vi "day 8 task 2.vi"() -> ()   [LabVIEW 2019]
panel:
  out "Input array":u8[][](array[numeric])
  out "each dir":i32[][][](array[numeric])
  out "multiplied together":i32[][](array[numeric])
  out "max value":i32
  # "up, left,right,down\nshould be\n1122\n\n2212\n\nnext try do by hand"
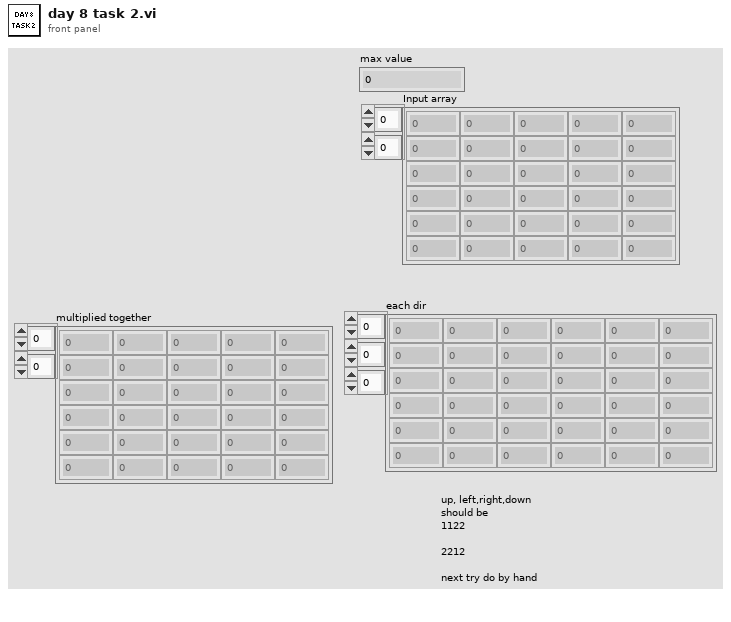
[diagram p1: front panel]
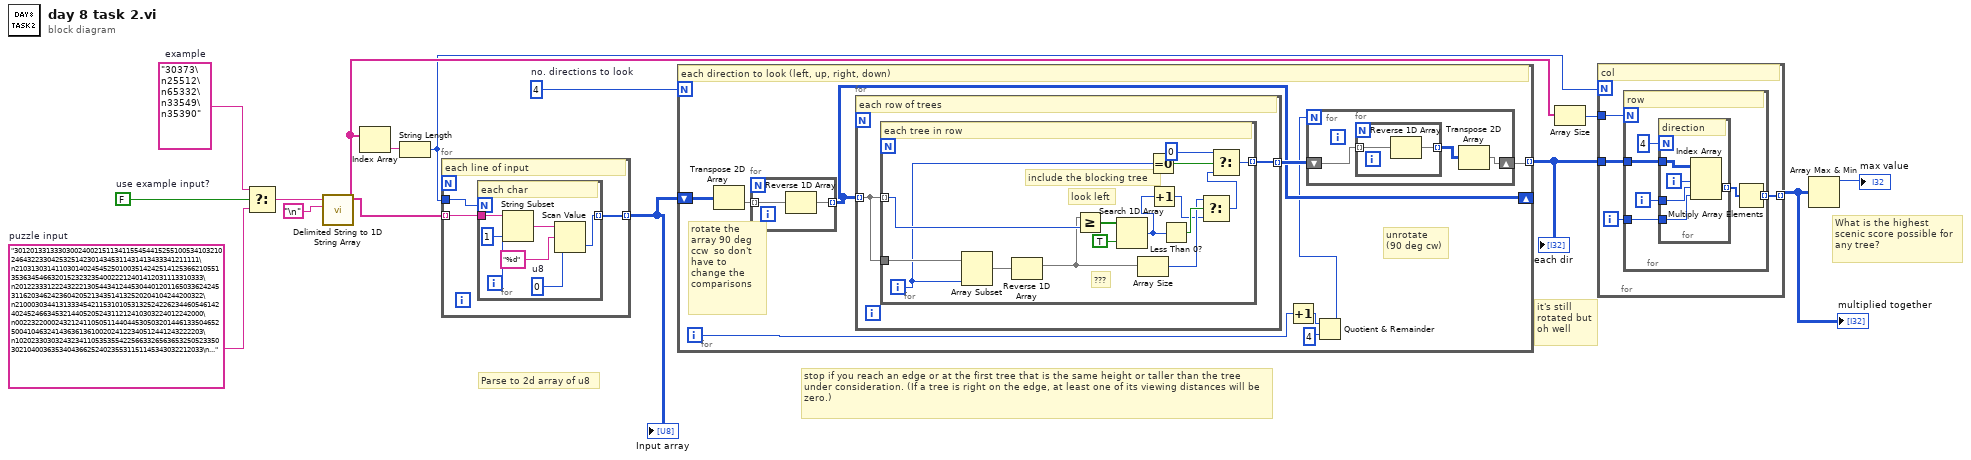
[diagram p0: block diagram]
diagram:
  w9 = 4  # no. directions to look
  w12 = "30373\n25512\n65332\n33549\n35390"  # example
  w13 = FALSE  # use example input?
  w14 = "301201331333030024002151134115545441525510053410321024643223304253251423014345311431413433341211111\n210313031411030140245452501003514242514125366210551353634546632015232323540022212401412031113310333\n201223331222432221305443412445304401201165033624245311620346242360420521343514132520204104244200322\n210003034413133345421153101053132524226234460546142402452466345321440520524311212410303224012242000\n002232200024321241105051144044530503201446133504652500410463241436361361002024122340512441243222203\n102023303032432341105353554225663326563653250523350302104003635340436625240235531151145343032212033\n..."  # puzzle input
  # "it's still\nrotated but\noh well"
  # "stop if you reach an edge or at the first tree that is the same height or taller than the tree under consideration. (If a tree is right on the edge, at least one of its viewing distances will be zero.)"
  # "What is the highest scenic score possible for any tree?"
  # "Parse to 2d array of u8"
  n1 = Select(t=w12, s=w13, f=w14) -> (s? t:f=w11:string)
  n2 = call <vilib>:"Delimited String to 1D String Array.vi"("delimiter"="\n", "delimited string"=w11) -> ("string array"=w2:string[])  [unwired: 9 in]
  n3 = Index Array(array=w2) -> (element=w8:string)  [unwired: 1 in]
  n4 = String Length(string=w8) -> (length=w1:i32)
  n5 = for {
    tunnel: w2 -> [w17] mode=indexing
    tunnel: [w16] -> w7 mode=indexing
    tunnel: w1 -> [w15]
    # "each line of input"
    n6 = for {
      N: w15 -> [_]
      tunnel: w17 -> [w24]
      tunnel: [w20] -> w16 mode=indexing
      i -> [w18]
      w21 = u8 0  # u8
      # "each char"
      n7 = String Subset(string=w24, offset (0)=w18, length (rest)=1 ("length (rest)")) -> (substring=w23:string)
      n8 = Scan Value(string=w23, format string="%d", default (0 dbl)=w21) -> (value=w20:u8)  [unwired: 1 out]
    }
  }
  "Input array" <- w7
  n9 = for {
    N: w9 -> [_]
    shift-right: [w29] -> _
    shift-left: w7 -> [w33]
    tunnel: [w32] -> w4 mode=indexing
    i -> [w26]
    # "unrotate\n(90 deg cw)"
    # "rotate the array 90 deg ccw  so don't have to change the comparisons"
    # "each direction to look (left, up, right, down)"
    n10 = Transpose 2D Array(2D array=w33) -> (transposed array=w30:u8[][])
    n11 = for {
      tunnel: w30 -> [w35] mode=indexing
      tunnel: [w34] -> w29 mode=indexing
      n12 = Reverse 1D Array(array=w35) -> (reversed array=w34:u8[])
    }
    n13 = for {
      tunnel: w29 -> [w42] mode=indexing
      tunnel: [w41] -> w31 mode=indexing
      # "each row of trees"
      n14 = for {
        tunnel: w42 -> [w52] mode=indexing
        tunnel: w42 -> [w57]
        tunnel: [w55] -> w41 mode=indexing
        i -> [w46]
        # "include the blocking tree"
        # "???"
        # "look left"
        # "each tree in row"
        n15 = Array Subset(array=w57, length=w46) -> (w43:u8[])  [unwired: 1 in]
        n16 = Reverse 1D Array(array=w43) -> (reversed array=w44:u8[])
        n17 = Greater Or Equal?(x=w44, y=w52) -> (x >= y?=w53:bool[])
        n18 = Search 1D Array(1D array=w53, element=TRUE) -> (index of element=w47:i32)  [unwired: 1 in]
        n19 = Array Size(array=w44) -> (size(s)=w49:i32)
        n20 = Equal To 0?(x=w46) -> (x = 0?=w56:bool)
        n21 = Increment(x=w47) -> (x+1=w48:i32)
        n22 = Less Than 0?(x=w47) -> (x < 0?=w50:bool)
        n23 = Select(t=w49, s=w50, f=w48) -> (s? t:f=w45:i32)
        n24 = Select(t=0, s=w56, f=w45) -> (s? t:f=w55:i32)
      }
    }
    n25 = Increment(x=w26) -> (x+1=w27:i32)
    n26 = Quotient & Remainder(x=w27, y=4) -> (x-y*floor(x/y)=w25:i32)  [unwired: 1 out]
    n27 = for {
      N: w25 -> [_]
      shift-right: [w36] -> w32
      shift-left: w31 -> [w38]
      n28 = for {
        tunnel: w38 -> [w40] mode=indexing
        tunnel: [w39] -> w37 mode=indexing
        n29 = Reverse 1D Array(array=w40) -> (reversed array=w39:i32[])
      }
      n30 = Transpose 2D Array(2D array=w37) -> (transposed array=w36:i32[][])
    }
  }
  "each dir" <- w4
  n31 = Array Size(array=w2) -> (size(s)=w3:i32)
  n32 = for {
    N: w1 -> [_]
    tunnel: w4 -> [w61]
    tunnel: [w59] -> w6 mode=indexing
    tunnel: w3 -> [w58]
    i -> [w60]
    # "col"
    n33 = for {
      N: w58 -> [_]
      tunnel: w61 -> [w67]
      tunnel: w60 -> [w65]
      tunnel: [w63] -> w59 mode=indexing
      i -> [w66]
      # "row"
      n34 = for {
        N: 4 -> [_]
        tunnel: w67 -> [w72]
        tunnel: [w71] -> w64 mode=indexing
        tunnel: w66 -> [w69]
        tunnel: w65 -> [w68]
        i -> [w70]
        # "direction"
        n35 = Index Array(array=w72, index (dim 0)=w70, index (dim 1)=w69, index (dim 2)=w68) -> (element=w71:i32)
      }
      n36 = Multiply Array Elements(1:w64) -> (0:w63:i32)
    }
  }
  "multiplied together" <- w6
  n37 = Array Max & Min(array=w6) -> (max value=→"max value":i32)  [unwired: 3 out]
